vi "disdrometer_2020_09_09.vi"(0 "Port":refnum<visa-resource-name>="Port2") -> ()   [LabVIEW 2018]
doc: "Logs and displays data in real-time from the Thies Clima Disdrometer."
uses:
  Distrometer_States.ctl
  disdrometer_MainClust.ctl
  Disdrometer_Message_To_Send_Enum.ctl
  Epimedia_Connex_Source/HDF5/DisdromterSummaryData.ctl
  Disdrometer_Status_Cluster.ctl
  Disdrometer_PlotData_Clust.ctl
  Disdrometer_UserDefined_clust.ctl
  Epimedia_Connex_Source/Controls/Enums/WatchdogTimer_Enum.ctl
  Epimedia_Connex_Source/Controls/Enums/LogLoopEnum.ctl
  Epimedia_Connex_Source/HDF5/DisdrometerData.ctl
panel:
  in  "Raw String File Path":path=path "C:/ConnexData"
  out "code":i32
  out "status":bool
  in  "AutoReset":bool=TRUE
  in  "SNR Threshold":dbl caption="Don't reset at 90 days if 84 Co peak amplitude is below this SNR Threshold (dBm)" format="%#_13g"
  in  "UserCommand":string="RS00001"
  in  "Submit":bool
  out "Sync Error":bool
  out "Sync String":string="Currently out of sync with Disdrometer.\nPolling at 5s delay until sync resumes."
  out "Poll Response:":string
  out "Observed":dbl
  out "Radar Reflectivity":dbl
  out "Visibility":dbl
  out "Uptime":string="00:00:00"
  out "Progress Bar":u32(slide) scale=0.0..60.0
  out "Interior Temp.":dbl
  out "Observed":dbl
  out "Accumulation":dbl
  out "Rain Rate":dbl
  in  "stop":bool
  out "Header":picture
  out "Velocity":cluster{dbl[], "Diameter Distribution":dbl[]}(graph)
  out "Size":cluster{dbl[], "Diameter Distribution":dbl[]}(graph)
  out "Accumulation":cluster{"Today":dbl[], "Today":dbl[]}(graph)
  out "Rain Rate":cluster{"Today":dbl[], "Today":dbl[]}(graph)
  # "v.20210913"
  # "INPUT / OUTPUT SETTINGS"
  # "CONDITIONS"
  # "(last 1 minute)"
  # "mm / hr"
  # "mm"
  # "particles"
  # "total particles"
  # "°C"
  # "m"
  # "dBz"
  # "Recording"
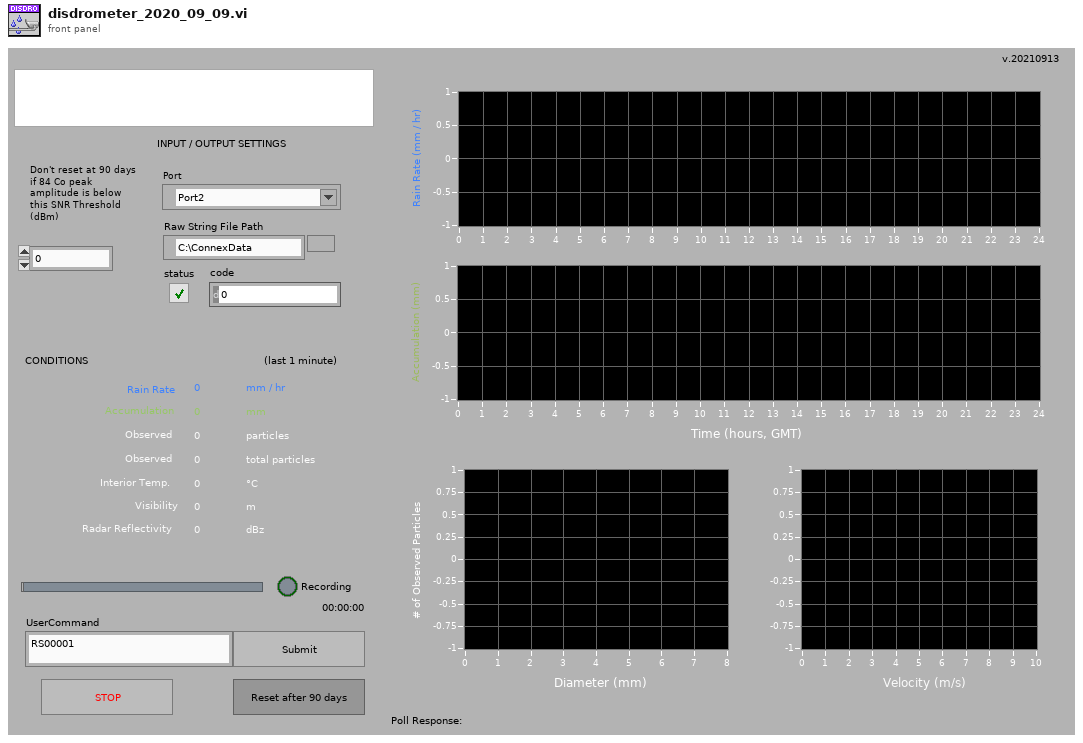
[diagram p1: front panel]
types:
  T1 = typedef "disdrometer_MainClust.ctl" = cluster{"Response":string, "ResetAccum":bool, "SyncErr":bool, "Enum":T2, "RainingNow":bool, "Parsed":T3, "Spectrum":dbl[], "DisdromStatus":T4, "Plot":T5, "User":T6}
  T2 = typedef "Disdrometer_Message_To_Send_Enum.ctl" = enum16{"None", "ResetAccum", "ResetDisdrom", "UserCommand"}
  T3 = typedef "DisdromterSummaryData.ctl" = cluster{"current time":dbl, "Timestamp":dbl, "Total Rain Rate":dbl, "Liquid Rain Rate":dbl, "Solid Rain Rate":dbl, "Total Rainfall":dbl, "Visibility":dbl, "Radar Reflectivity":dbl, "Max Diameter Hail":dbl, "Measured Particles":i32, "Particle Min Speed":i16, "Particle Max Speed":i16, "Particle Min Diam":i16, "NonHydr Particles":i16, "NonHydr Volume":dbl, "Unkn Particles":i16, "Unkn Volume":dbl, "HydroType":i8}
  T4 = typedef "Disdrometer_Status_Cluster.ctl" = cluster{"Laser":bool, "Signal":bool, "LaserTemp_Analog":bool, "LaserTemp_Digital":bool, "LaserCurrent_Analog":bool, "LaserCurrent_Digital":bool, "SensorSupply":bool, "HeatLaserHead":bool, "HeatReceiverHead":bool, "TempSensor":bool, "HeatSupply":bool, "HeatHousing":bool, "HeatHeads":bool, "HeatCarriers":bool, "OutputLaserPower":bool, "Checksum":bool, "StatusInt":u16}
  T5 = typedef "Disdrometer_PlotData_Clust.ctl" = cluster{"SizeDistrib":dbl[], "VelocityDistrib":dbl[], "Today":dbl[][], "Yesterday":dbl[][]}
  T6 = typedef "Disdrometer_UserDefined_clust.ctl" = cluster{"Port":refnum<visa-resource-name>, "SNR Threshold":dbl, "FileFolder":path}
  T7 = typedef "Distrometer_States.ctl" = enum16{"Disdr_Init", "Disdr_ChkTime", "Disdr_Read", "Disdr_Parse"}
  T8 = typedef "WatchdogTimer_Enum.ctl" = enum16{"ResetAll", "CheckAll", "HW1", "HW2", "Tones", "FP", "Noise", "Log", "TCP", "AI", "TC", "ADAM", "Disdrom", "TE", "Weather"}
  T9 = typedef "DisdrometerData.ctl" = cluster{"Spectrum Data":i16[], "DisdromSummary":T3, "Status":T4}
  T10 = typedef "LogLoopEnum.ctl" = enum16{"Log_Init", "Log_Config", "Log_CfgAlarm", "Log_TimeDomain", "Log_Tone", "Log_NoiseTrace", "Log_NoiseSum", "Log_DO", "Log_AI", "Log_TC", "Log_Disdrom", "Log_Weather", "Log_TE", "Log_ADAM", "Log_UPS", "Log_ChkTime", "Log_Alarm", "Log_SSH", "Log_Write", "Log_Exit"}
  T11 = cluster{"[0]":dbl, "[1]":dbl, "[2]":dbl, "[3]":dbl, "[4]":dbl, "[5]":dbl}
  T12 = typedef "imagedata.ctl" = cluster{"image type":i32, "image depth":i32, "image":u8[], "mask":u8[], "colors":u32[], "Rectangle":cluster{"left":i16, "top":i16, "right":i16, "bottom":i16}}
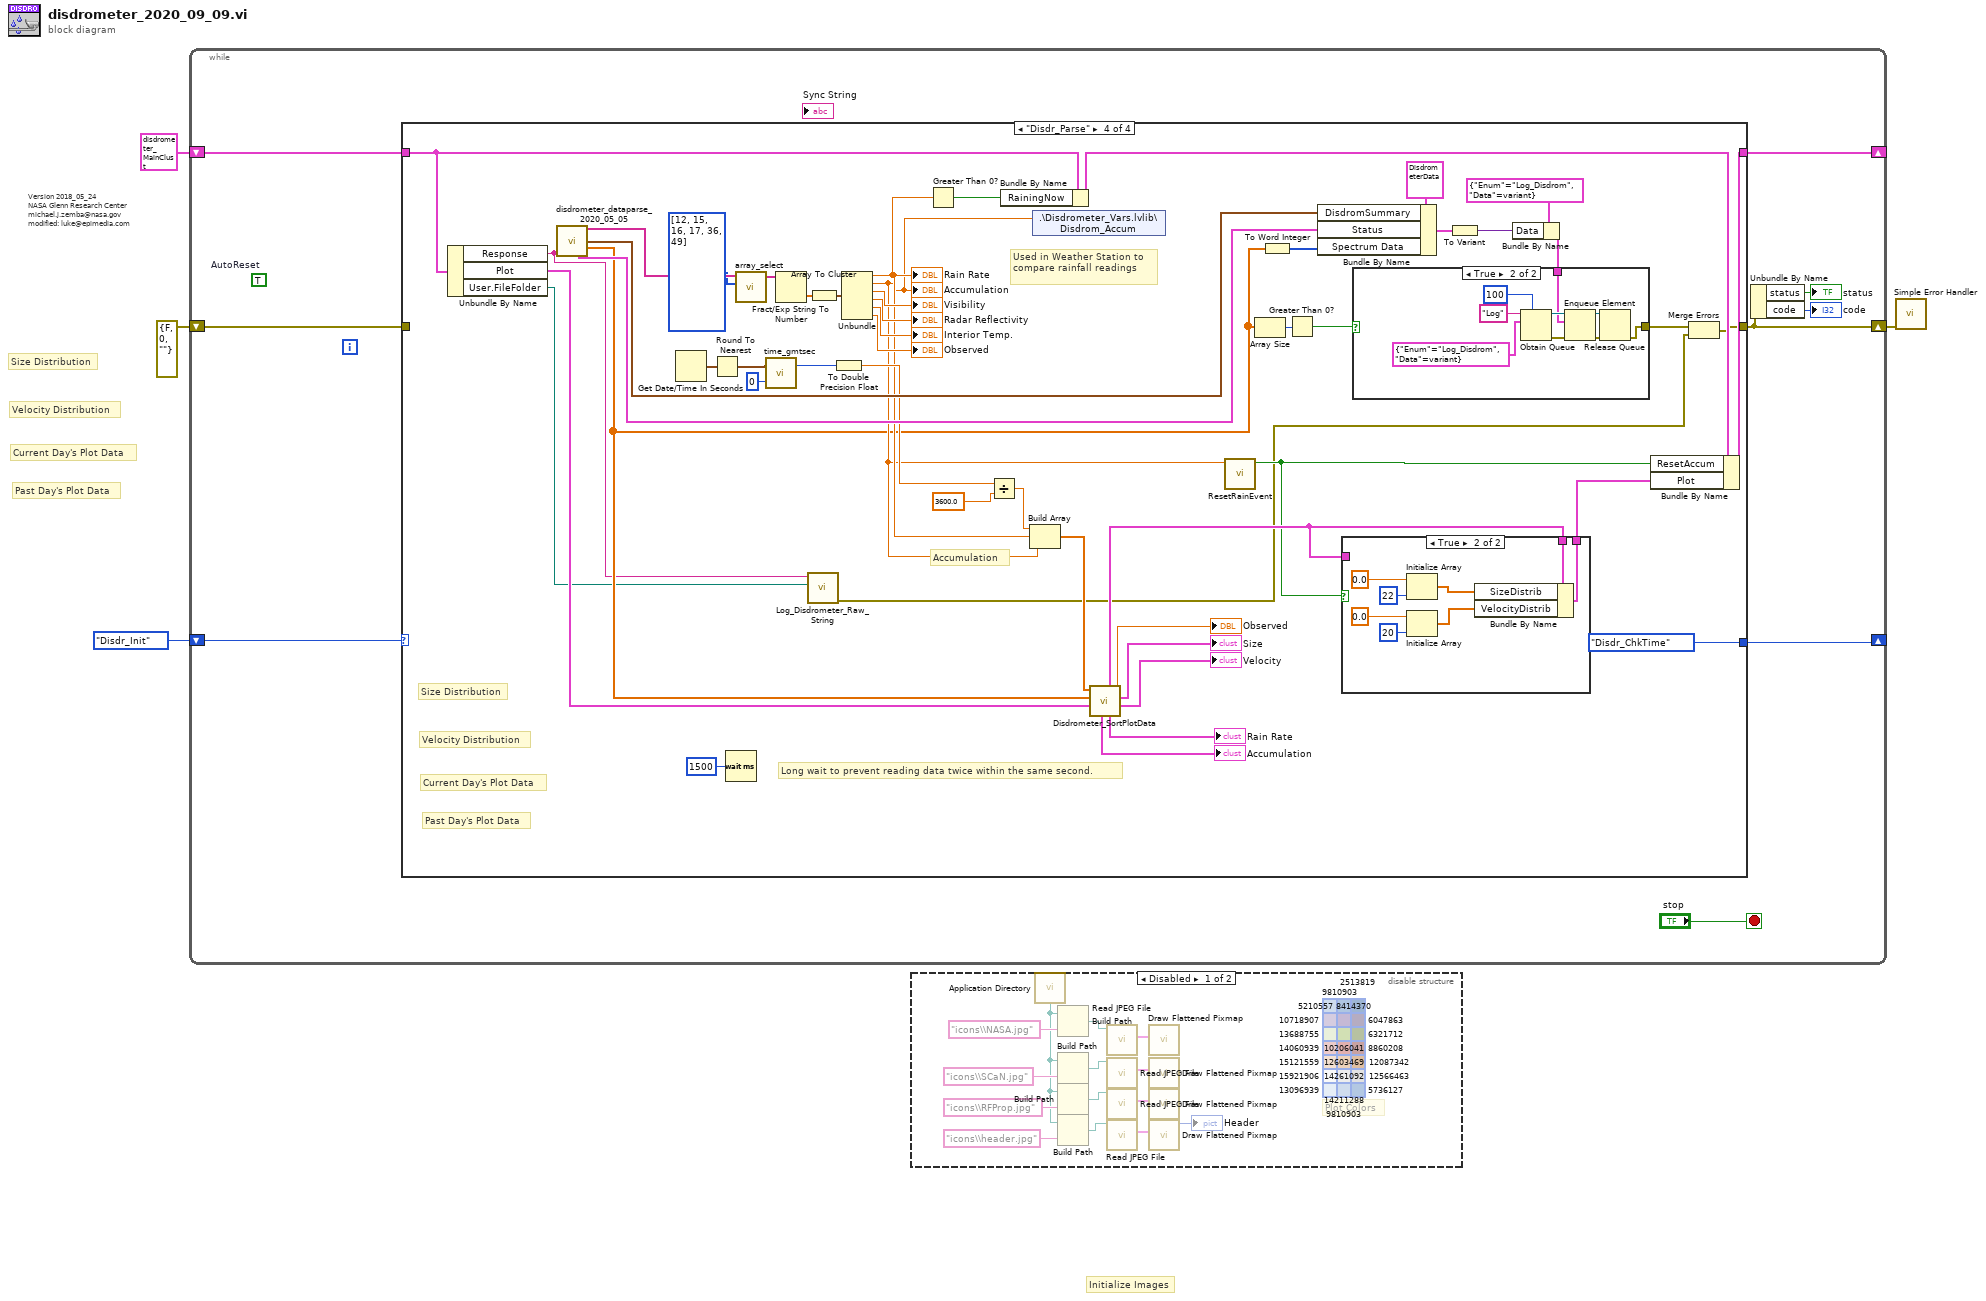
[diagram p0: block diagram]
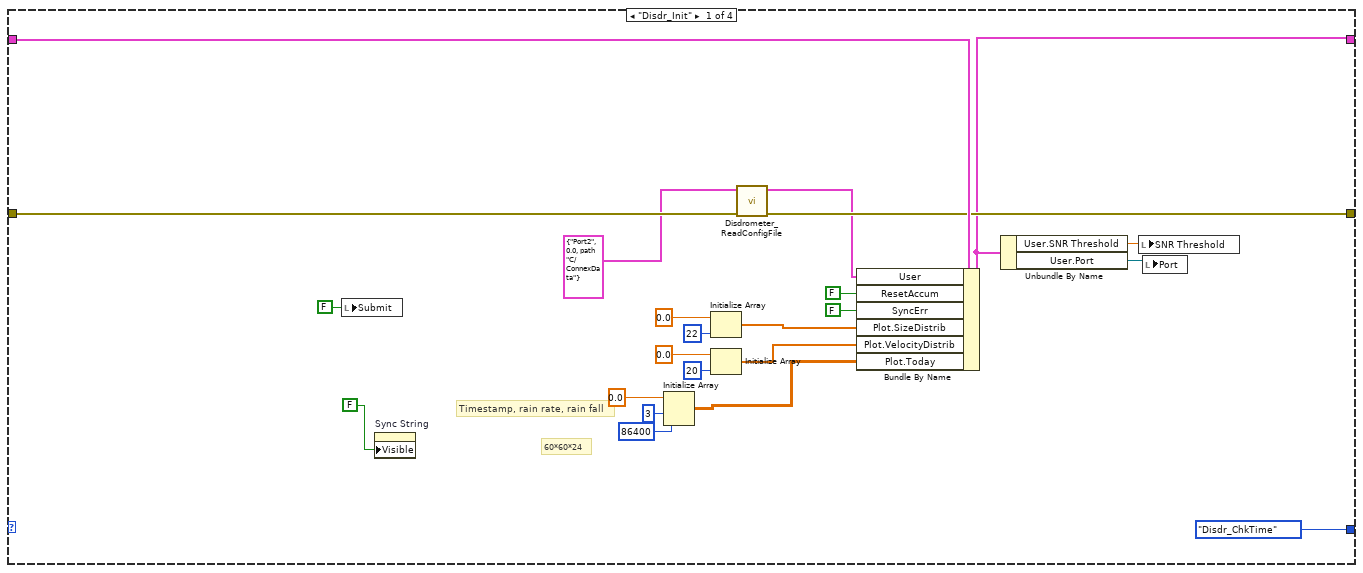
[diagram p3: hidden frame]
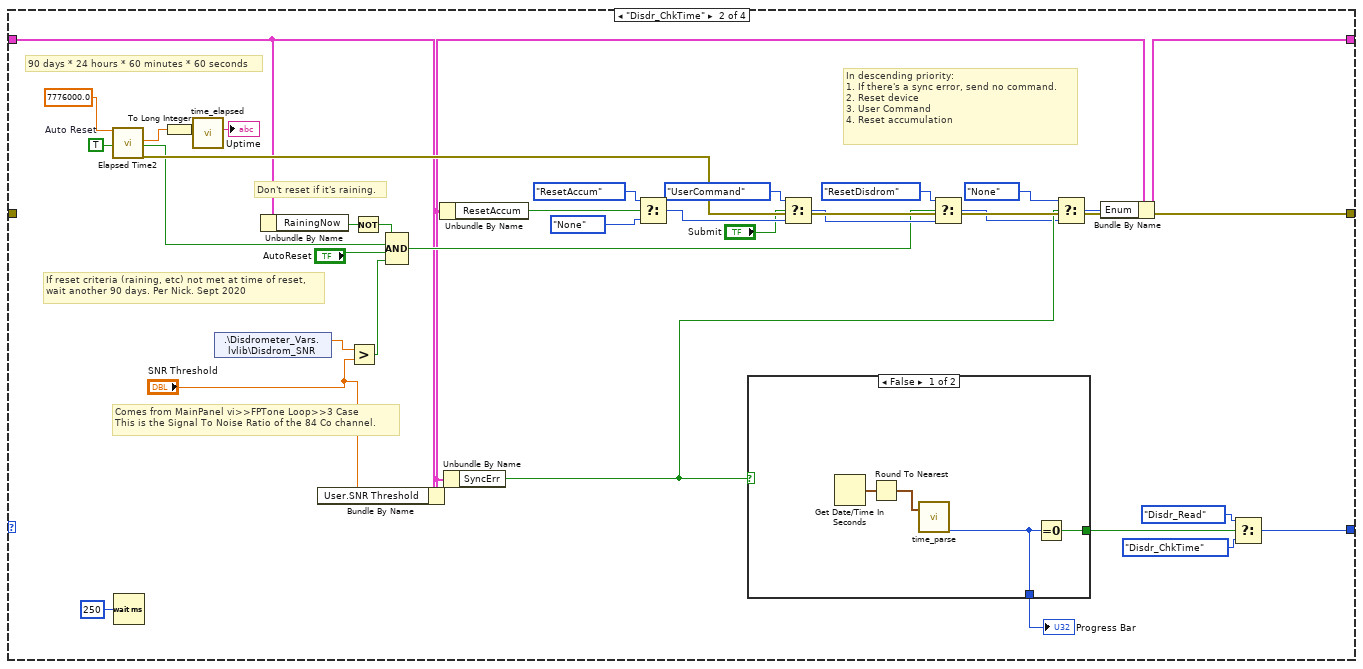
[diagram p4: hidden frame]
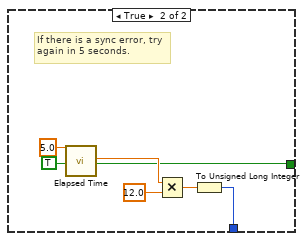
[diagram p5: hidden frame]
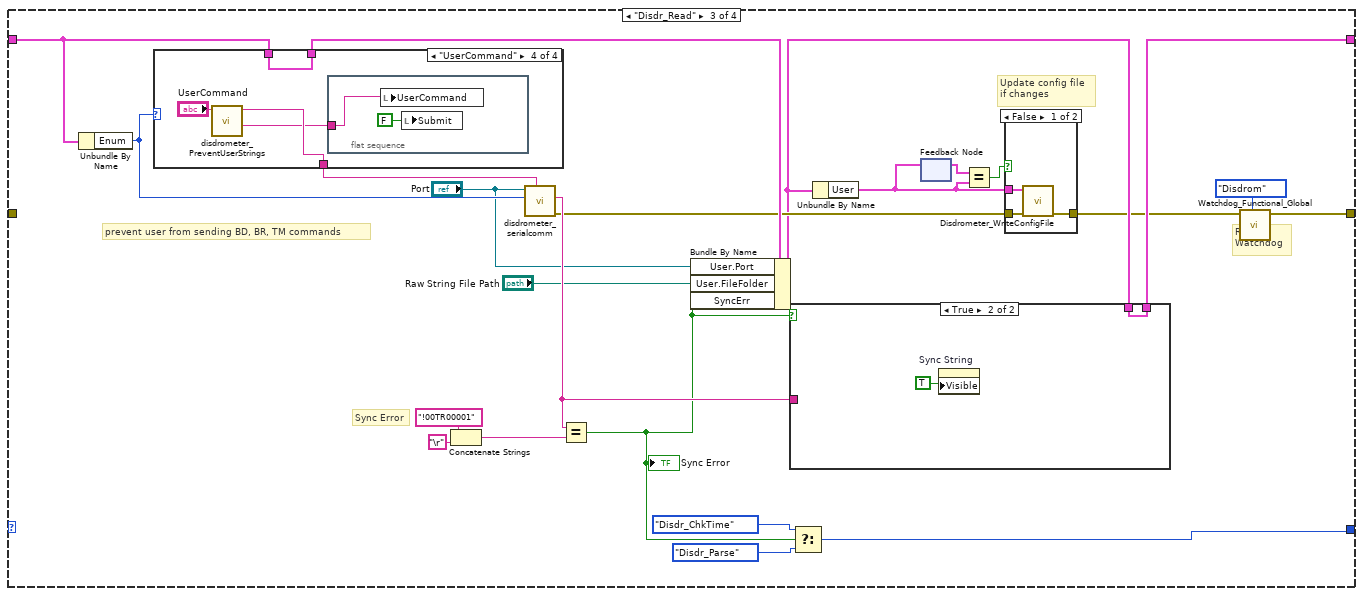
[diagram p6: hidden frame]
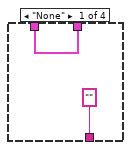
[diagram p8: hidden frame]
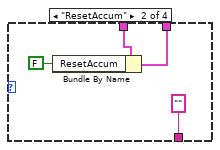
[diagram p9: hidden frame]
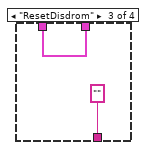
[diagram p10: hidden frame]
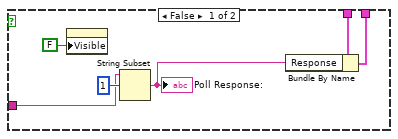
[diagram p11: hidden frame]
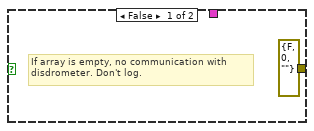
[diagram p12: hidden frame]
diagram:
  # "Version 2018_05_24\nNASA Glenn Research Center\nmichael.j.zemba@nasa.gov\nmodified: luke@epimedia.com"
  # "Past Day's Plot Data"
  # "Current Day's Plot Data"
  # "Velocity Distribution"
  # "Size Distribution"
  # "Initialize Images"
  n1 = while {
    shift-right: [w7] -> w4
    shift-left: errorcluster {"status"=FALSE, "code"=0, "source"=""} ("error out") -> [w9]
    shift-right: [w11] -> _
    shift-left: Distrometer_States."Disdr_Init" -> [w12]
    shift-right: [w10] -> _
    shift-left: T1 {"Response"="", "ResetAccum"=FALSE, "SyncErr"=FALSE, "Enum"=enum."ResetAccum", "RainingNow"=FALSE, "Parsed"={"current time"=0.0, "Timestamp"=0.0, "Total Rain Rate"=0.0, "Liquid Rain Rate"=0.0, "Solid Rain Rate"=0.0, "Total Rainfall"=0.0, "Visibility"=0.0, "Radar Reflectivity"=0.0, "Max Diameter Hail"=0.0, "Measured Particles"=0, "Particle Min Speed"=0, "Particle Max Speed"=0, "Particle Min Diam"=0, "NonHydr Particles"=0, "NonHydr Volume"=0.0, "Unkn Particles"=0, "Unkn Volume"=0.0, "HydroType"=0}, "Spectrum"=[], "DisdromStatus"={"Laser"=TRUE, "Signal"=TRUE, "LaserTemp_Analog"=TRUE, "LaserTemp_Digital"=TRUE, "LaserCurrent_Analog"=TRUE, "LaserCurrent_Digital"=TRUE, "SensorSupply"=TRUE, "HeatLaserHead"=TRUE, "HeatReceiverHead"=TRUE, "TempSensor"=TRUE, "HeatSupply"=TRUE, "HeatHousing"=TRUE, "HeatHeads"=TRUE, "HeatCarriers"=TRUE, "OutputLaserPower"=TRUE, "Checksum"=TRUE, "StatusInt"=0}, "Plot"={"SizeDistrib"=[], "VelocityDistrib"=[], "Today"=[], "Yesterday"=[]}, "User"={"Port"="Port2", "SNR Threshold"=0.0, "FileFolder"=path "C:/ConnexData"}} -> [w8]
    stop <- "stop" stop-if-true
    (unwired) TRUE  # AutoReset
    n2 = case shown="\"Disdr_Parse\"" w12 {
      tunnel: [w20 w64 w83 w133] -> w7
      tunnel: [Distrometer_States."Disdr_ChkTime" w69 w98 Distrometer_States."Disdr_ChkTime"] -> w11
      tunnel: [w16 w62 w101 w170] -> w10
      tunnel: w8 -> [w33 w43 w94 w141]
      tunnel: w9 -> [w19 _ _ _]
      frame "Disdr_Init" {
        # "Timestamp, rain rate, rain fall"
        # "60*60*24"
        n3 = local write "Submit"(FALSE ("Submit")) -> ()
        n4 = property on="Sync String" class="Str"("Visible"=FALSE) -> ()  [unwired: 2 in, 2 out]
        n5 = Initialize Array(0.0, 3 ("dimension size"), 86400 ("dimension size")) -> (w22:dbl[][])
        n6 = Initialize Array(0.0, 22 ("dimension size")) -> (w27:dbl[])
        n7 = Initialize Array(0.0, 20 ("dimension size")) -> (w26:dbl[])
        n8 = call "Disdrometer_ReadConfigFile.vi"("ErrorIn"=w19, "User"=T6 {"Port"="Port2", "SNR Threshold"=0.0, "FileFolder"=path "C:/ConnexData"}) -> ("ErrorOut"=w20:errorcluster, "User"=w17:T6)  [unwired: 7 in, 1 out]
        n9 = Bundle By Name(cluster=w33, "User"=w17, "ResetAccum"=FALSE, "SyncErr"=FALSE ("SyncStatus"), "Plot.SizeDistrib"=w27, "Plot.VelocityDistrib"=w26, "Plot.Today"=w22) -> (w16:T1)
        n10 = Unbundle By Name(w16) -> ("User.SNR Threshold"=w15:dbl, "User.Port"=w14:refnum<visa-resource-name>)
        n11 = local write "SNR Threshold"(w15) -> ()
        n12 = local write "Port"(w14) -> ()
      }
      frame "Disdr_ChkTime" {
        w41 = TRUE  # Auto Reset
        # "If reset criteria (raining, etc) not met at time of reset, \nwait another 90 days. Per Nick. Sept 2020"
        # "Comes from MainPanel vi>>FPTone Loop>>3 Case\nThis is the Signal To Noise Ratio of the 84 Co channel."
        # "Don't reset if it's raining."
        # "90 days * 24 hours * 60 minutes * 60 seconds"
        # "In descending priority:\n1. If there's a sync error, send no command.\n2. Reset device\n3. User Command\n4. Reset accumulation"
        n13 = call "Elapsed Time2"("Time Target (s)"=7776000.0 ("x"), "Auto Reset"=w41) -> ("Elapsed Time (s)"=w51:dbl, "Time has Elapsed"=w39:bool, "error out"=w64:errorcluster)  [unwired: 10 in, 5 out]
        n14 = Wait (ms)(milliseconds to wait=u32 250) -> ()  [unwired: 1 out]
        n15 = To Long Integer(number=w51) -> (32bit integer=w63:i32)
        n16 = call "time_elapsed.vi"("Elapsed Time (sec)"=w63) -> ("Elapsed Time (string)"=→"Uptime":string)  [unwired: 10 in]
        n17 = shared-variable ".\\Disdrometer_Vars.lvlib\\Disdrom_SNR"() -> (w45:dbl)  [unwired: 1 in, 1 out]
        n18 = Unbundle By Name(w43) -> ("RainingNow"=w48:bool)
        n19 = Bundle By Name(cluster=w43, "User.SNR Threshold"="SNR Threshold") -> (w44:T1)
        n20 = Greater?(x=w45, y="SNR Threshold") -> (0:w38:bool)
        n21 = Not(x=w48) -> (.not. x?=w46:bool)
        n22 = Compound Arithmetic op=AND(w46, w39, "AutoReset", w38) -> (w47:bool)
        n23 = Unbundle By Name(w44) -> ("ResetAccum"=w49:bool)
        n24 = Unbundle By Name(w44) -> ("SyncErr"=w59:bool)
        n25 = Select(t=Disdrometer_Message_To_Send_Enum."ResetAccum" ("Enum"), s=w49, f=Disdrometer_Message_To_Send_Enum."None" ("Enum")) -> (s? t:f=w53:T2)
        n26 = case shown="False" w59 {
          tunnel: [w72 w80] -> w71
          tunnel: [w73 w78] -> w70
          frame False {
            n27 = Get Date/Time In Seconds() -> (seconds since 1Jan1904=w74:timestamp)
            n28 = Round To Nearest(number=w74) -> (nearest integer value=w75:timestamp)
            n29 = call "time_parse.vi"("Current Time"=w75) -> ("Seconds"=w72:u32)  [unwired: 12 in, 6 out]
            n30 = Equal To 0?(x=w72) -> (x = 0?=w73:bool)
          }
          frame True {
            # "If there is a sync error, try\nagain in 5 seconds."
            n31 = call "Elapsed Time"("Time Target (s)"=5.0, "Auto Reset"=TRUE) -> ("Elapsed Time (s)"=w82:dbl, "Time has Elapsed"=w78:bool)  [unwired: 10 in, 6 out]
            n32 = Multiply(x=w82, y=12.0) -> (x*y=w81:dbl)
            n33 = To Unsigned Long Integer(number=w81) -> (unsigned 32bit integer=w80:u32)
          }
        }
        "Progress Bar" <- w71
        n34 = Select(t=Disdrometer_Message_To_Send_Enum."UserCommand" ("Enum"), s="Submit", f=w53) -> (s? t:f=w55:T2)
        n35 = Select(t=Disdrometer_Message_To_Send_Enum."ResetDisdrom" ("Enum"), s=w47, f=w55) -> (s? t:f=w57:T2)
        n36 = Select(t=Disdrometer_Message_To_Send_Enum."None" ("Enum"), s=w59, f=w57) -> (s? t:f=w60:T2)
        n37 = Bundle By Name(cluster=w44, "Enum"=w60) -> (w62:T1)
        n38 = Select(t=Distrometer_States."Disdr_Read", s=w70, f=Distrometer_States."Disdr_ChkTime") -> (s? t:f=w69:T7)
      }
      frame "Disdr_Read" {
        # "Reset\nWatchdog"
        # "Update config file\nif changes"
        # "prevent user from sending BD, BR, TM commands"
        # "Sync Error"
        n39 = Unbundle By Name(w94) -> ("Enum"=w96:T2)
        n40 = case shown="\"UserCommand\"" w96 {
          tunnel: w94 -> [w111 w115 w117 w121]
          tunnel: [w111 w114 w117 w121] -> w95
          tunnel: ["" ("UserCommand") "" ("UserCommand") "" ("UserCommand") w119] -> w93
          frame "None" {
          }
          frame "ResetAccum" {
            n41 = Bundle By Name(cluster=w115, "ResetAccum"=FALSE) -> (w114:T1)
          }
          frame "ResetDisdrom" {
          }
          frame "UserCommand" {
            n42 = call "disdrometer_PreventUserStrings.vi"("UserCommand"="UserCommand") -> ("UserMessage"=w118:string, "Filtered Command"=w119:string)  [unwired: 8 in, 1 out]
            n43 = flat-sequence {
              tunnel: w118 -> [w122]
              frame #0 {
                n44 = local write "UserCommand"(w122) -> ()
                n45 = local write "Submit"(FALSE ("Submit")) -> ()
              }
            }
          }
        }
        n46 = Concatenate Strings("!00TR00001" ("x"), "\r") -> (w102:string)
        n47 = call "disdrometer_serialcomm.vi"("UserCommand"=w93, "CommandToSend"=w96, "Resource Name"="Port") -> ("Error Out"=w91:errorcluster, "Poll Response"=w105:string)  [unwired: 6 in, 1 out]
        n48 = Equal?(x=w105, y=w102) -> (x = y?=w97:bool)
        "Sync Error" <- w97
        n49 = Bundle By Name(cluster=w95, "User.Port"="Port", "User.FileFolder"="Raw String File Path", "SyncErr"=w97) -> (w90:T1)
        n50 = case shown="True" w97 {
          tunnel: w105 -> [w127 _]
          tunnel: w90 -> [w125 w130]
          tunnel: [w124 w130] -> w101
          frame False {
            n51 = property on="Sync String" class="Str"("Visible"=FALSE) -> ()  [unwired: 2 in, 2 out]
            n52 = String Subset(string=w127, offset (0)=1) -> (substring=w126:string)  [unwired: 1 in]
            "Poll Response:" <- w126
            n53 = Bundle By Name(cluster=w125, "Response"=w126) -> (w124:T1)
          }
          frame True {
            n54 = property on="Sync String" class="Str"("Visible"=TRUE) -> ()  [unwired: 2 in, 2 out]
          }
        }
        n55 = Select(t=Distrometer_States."Disdr_ChkTime", s=w97, f=Distrometer_States."Disdr_Parse") -> (s? t:f=w98:T7)
        n56 = Unbundle By Name(w90) -> ("User"=w88:T6)
        n57 = feedback-in #1(w88) -> ()
        n58 = feedback #1() -> (w89:T6)  [unwired: 1 in]
        n59 = Equal?(x=w89, y=w88) -> (x = y?=w87:bool)
        n60 = case shown="False" w87 {
          tunnel: w91 -> [w108 w109]
          tunnel: [w107 w109] -> w84
          tunnel: w88 -> [w106 _]
          frame False {
            n61 = call "Disdrometer_WriteConfigFile.vi"("ErrorIn"=w108, "User"=w106) -> ("ErrorOut"=w107:errorcluster)  [unwired: 9 in]
          }
          frame True {
          }
        }
        n62 = call "Watchdog_Functional_Global.vi"("Watchdog"=WatchdogTimer_Enum."Disdrom", "error in"=w84) -> ("error out"=w83:errorcluster)  [unwired: 8 in, 1 out]
      }
      frame "Disdr_Parse" {
        # "Used in Weather Station to compare rainfall readings"
        # "Long wait to prevent reading data twice within the same second."
        # "Accumulation"
        # "Past Day's Plot Data"
        # "Current Day's Plot Data"
        # "Velocity Distribution"
        # "Size Distribution"
        n63 = Unbundle By Name(w141) -> ("Response"=w134:string, "Plot"=w152:T5, "User.FileFolder"=w135:path)
        n64 = call "disdrometer_dataparse_2020_05_05.vi"("Poll Response"=w134) -> ("Complete Dataset"=w178:string[], "output cluster"=w177:T3, "Spectrum Data"=w138:dbl[], "DisdromStatus"=w176:T4)  [unwired: 11 in]
        n65 = Get Date/Time In Seconds() -> (seconds since 1Jan1904=w174:timestamp)
        n66 = Round To Nearest(number=w174) -> (nearest integer value=w173:timestamp)
        n67 = Wait (ms)(milliseconds to wait=u32 1500) -> ()  [unwired: 1 out]
        n68 = call "array_select.vi"("Selection"=i32[] [12, 15, 16, 17, 36, 49], "Array In"=w178) -> ("Array Out"=w169:string[])  [unwired: 9 in]
        n69 = call "time_gmtsec.vi"("Timezone Offset (Hrs)"=0, "Timestamp"=w173) -> ("Sec Since 12AM GMT"=w175:u32)  [unwired: 1 out]
        n70 = Fract/Exp String To Number(string=w169) -> (number=w168:dbl[])  [unwired: 3 in, 1 out]
        n71 = call "Log_Disdrometer_Raw_String.vi"("FileFolder"=w135, "Response"=w134) -> ("error out"=w132:errorcluster)  [unwired: 9 in]
        n72 = Array To Cluster(array=w168) -> (cluster=w167:T11)
        n73 = To Double Precision Float(number=w175) -> (double precision float=w171:dbl)
        n74 = Unbundle(w167) -> ("[0]"=w143:dbl, "[1]"=w139:dbl, "[2]"=→"Visibility":dbl, "[3]"=→"Radar Reflectivity":dbl, "[4]"=→"Interior Temp.":dbl, "[5]"=→"Observed":dbl)
        "Rain Rate" <- w143
        "Accumulation" <- w139
        n75 = Greater Than 0?(x=w143) -> (x > 0?=w140:bool)
        n76 = Divide(x=w171, y=3600.0) -> (x/y=w165:dbl)
        n77 = Bundle By Name(cluster=w141, "RainingNow"=w140) -> (w142:T1)
        n78 = Build Array(w165, w143, w139) -> (w180:dbl[])
        n79 = shared-variable ".\\Disdrometer_Vars.lvlib\\Disdrom_Accum"(w139) -> ()  [unwired: 1 in, 1 out]
        n80 = call "Disdrometer_SortPlotData.vi"("Plot Data"=w152, "Spectrum"=w138, "Time, Rate, Accum"=w180) -> ("Velocity"=→"Velocity":cluster{dbl[], "Diameter Distribution":dbl[]}, "Size"=→"Size":cluster{dbl[], "Diameter Distribution":dbl[]}, "Observed"=→"Observed":dbl, "Rain Rate"=→"Rain Rate":cluster{"Today":dbl[], "Today":dbl[]}, "Plot out"=w146:T5, "Accumulation"=→"Accumulation":cluster{"Today":dbl[], "Today":dbl[]})  [unwired: 3 in]
        n81 = call "ResetRainEvent.vi"("RainAccumulation"=w139) -> ("Time has Elapsed"=w144:bool)  [unwired: 9 in, 1 out]
        n82 = Array Size(array=w138) -> (size(s)=w137:i32)
        n83 = To Word Integer(number=w138) -> (16bit integer=w154:i16[])
        n84 = Greater Than 0?(x=w137) -> (x > 0?=w136:bool)
        n85 = Bundle By Name(cluster=T9 {"Spectrum Data"=[], "DisdromSummary"={"current time"=0.0, "Timestamp"=0.0, "Total Rain Rate"=0.0, "Liquid Rain Rate"=0.0, "Solid Rain Rate"=0.0, "Total Rainfall"=0.0, "Visibility"=0.0, "Radar Reflectivity"=0.0, "Max Diameter Hail"=0.0, "Measured Particles"=0, "Particle Min Speed"=0, "Particle Max Speed"=0, "Particle Min Diam"=0, "NonHydr Particles"=0, "NonHydr Volume"=0.0, "Unkn Particles"=0, "Unkn Volume"=0.0, "HydroType"=0}, "Status"={"Laser"=TRUE, "Signal"=TRUE, "LaserTemp_Analog"=TRUE, "LaserTemp_Digital"=TRUE, "LaserCurrent_Analog"=TRUE, "LaserCurrent_Digital"=TRUE, "SensorSupply"=TRUE, "HeatLaserHead"=TRUE, "HeatReceiverHead"=TRUE, "TempSensor"=TRUE, "HeatSupply"=TRUE, "HeatHousing"=TRUE, "HeatHeads"=TRUE, "HeatCarriers"=TRUE, "OutputLaserPower"=TRUE, "Checksum"=TRUE, "StatusInt"=0}}, "DisdromSummary"=w177, "Status"=w176, "Spectrum Data"=w154) -> (w159:T9)
        n86 = case shown="True" w144 {
          tunnel: w146 -> [_ _]
          tunnel: w146 -> [w192 w194]
          tunnel: [w192 w193] -> w145
          frame False {
          }
          frame True {
            n87 = Initialize Array(0.0, 22 ("dimension size")) -> (w196:dbl[])
            n88 = Initialize Array(0.0, 20 ("dimension size")) -> (w195:dbl[])
            n89 = Bundle By Name(cluster=w194, "SizeDistrib"=w196, "VelocityDistrib"=w195) -> (w193:T5)
          }
        }
        n90 = To Variant(anything=w159) -> (Variant=w163:variant)
        n91 = Bundle By Name(cluster=cluster{"Enum":T10, "Data":variant} {"Enum"=enum."Log_Disdrom", "Data"=variant}, "Data"=w163) -> (w161:cluster{"Enum":T10, "Data":variant})
        n92 = case shown="True" w136 {
          tunnel: [errorcluster {"status"=FALSE, "code"=0, "source"=""} ("error out") w191] -> w181
          tunnel: w161 -> [_ w186]
          frame False {
            # "If array is empty, no communication with \ndisdrometer. Don't log."
          }
          frame True {
            n93 = Obtain Queue(max queue size (-1, unlimited)=100, name (unnamed)="Log", element data type=cluster{"Enum":T10, "Data":variant} {"Enum"=enum."Log_Disdrom", "Data"=variant}) -> (queue out=w188:refnum<queue>, error out=w187:errorcluster)  [unwired: 2 in, 1 out]
            n94 = Enqueue Element(queue=w188, element=w186, error in (no error)=w187) -> (queue out=w185:refnum<queue>, error out=w184:errorcluster)  [unwired: 1 in, 1 out]
            n95 = Release Queue(queue=w185, error in (no error)=w184) -> (error out=w191:errorcluster)  [unwired: 1 in, 2 out]
          }
        }
        n96 = Bundle By Name(cluster=w142, "ResetAccum"=w144, "Plot"=w145) -> (w170:T1)
        n97 = Merge Errors(w181, w132) -> (w133:errorcluster)
      }
    }
    n98 = Unbundle By Name(w7) -> ("status"=→"status":bool, "code"=→"code":i32)
  }
  n99 = disable-structure shown="Disabled" {
    frame Disabled {
      (unwired) u32 6321712
      (unwired) u32 8860208
      (unwired) u32 12087342
      (unwired) u32 12566463
      (unwired) u32 5736127
      (unwired) u32 14060939
      (unwired) u32 15121559
      (unwired) u32 15921906
      (unwired) u32 13096939
      (unwired) u32 13688755
      (unwired) u32 6047863
      (unwired) u32 10718907
      (unwired) u32 9810903
      (unwired) u32 10206041
      (unwired) u32 8414370
      (unwired) u32 12603469
      (unwired) u32 14261092
      (unwired) u32 14211288
      (unwired) u32 9810903
      (unwired) u32 2513819
      (unwired) u32 5210557
      # "Plot Colors"
      n100 = call <vilib>:"Application Directory.vi"() -> ("Application Directory"=w201:path)
      n101 = Build Path(base path=w201, name or relative path="icons\\NASA.jpg") -> (appended path=w212:path)
      n102 = Build Path(base path=w201, name or relative path="icons\\SCaN.jpg") -> (appended path=w211:path)
      n103 = Build Path(base path=w201, name or relative path="icons\\RFProp.jpg") -> (appended path=w208:path)
      n104 = Build Path(base path=w201, name or relative path="icons\\header.jpg") -> (appended path=w202:path)
      n105 = call <vilib>:"Read JPEG File.vi"("path to JPEG file"=w212) -> ("image data"=w216:T12)  [unwired: 8 in, 2 out]
      n106 = call <vilib>:"Read JPEG File.vi"("path to JPEG file"=w211) -> ("image data"=w215:T12)  [unwired: 8 in, 2 out]
      n107 = call <vilib>:"Read JPEG File.vi"("path to JPEG file"=w208) -> ("image data"=w210:T12)  [unwired: 8 in, 2 out]
      n108 = call <vilib>:"Read JPEG File.vi"("path to JPEG file"=w202) -> ("image data"=w207:T12)  [unwired: 8 in, 2 out]
      n109 = call <vilib>:"Draw Flattened Pixmap.vi"("image data"=w216) -> ()  [unwired: 8 in, 1 out]
      n110 = call <vilib>:"Draw Flattened Pixmap.vi"("image data"=w215) -> ("new picture"=w205:picture)  [unwired: 8 in]
      n111 = call <vilib>:"Draw Flattened Pixmap.vi"("image data"=w210) -> ("new picture"=w204:picture)  [unwired: 8 in]
      n112 = call <vilib>:"Draw Flattened Pixmap.vi"("image data"=w207) -> ("new picture"=→"Header":picture)  [unwired: 8 in]
    }
    frame Enabled {
    }
  }
  n113 = call <vilib>:"Simple Error Handler.vi"("error in (no error)"=w4) -> ()  [unwired: 1 in, 8 out]
